vi "File_Update a Path in Keeper.vi"(8 "Error":errorcluster, 9 "File / Directory Name":string, 10 "New Path":path, 11 "INI File Path":path) -> (0 "Error Out":errorcluster)   [LabVIEW 2020]
uses:
  <vilib>/Utility/config.llb/NI_LVConfig.lvlib
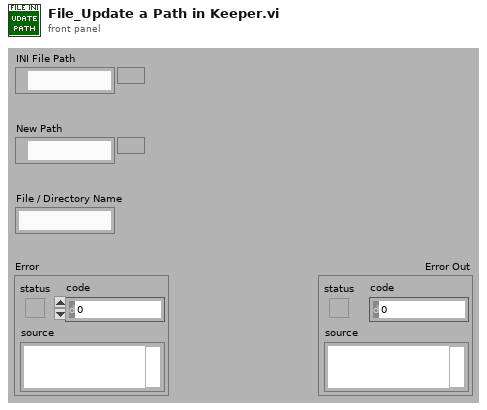
[diagram p1: front panel]
types:
  T1 = typedef "NI_LVConfig.lvlib/Config Data RefNum.ctl" = refnum<k1>
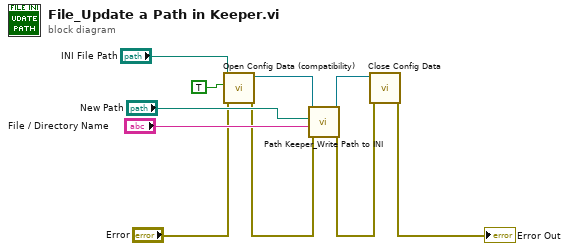
[diagram p0: block diagram]
diagram:
  n1 = call <vilib>:"Open Config Data (compatibility).vi"("error in (no error)"="Error", "create file if necessary (T)"=TRUE ("create file if necessary? (T)"), "configuration file path"="INI File Path") -> ("error out"=w5:errorcluster, "refnum"=w7:T1)  [unwired: 6 in, 1 out]
  n2 = call "Path Keeper_Write Path to INI.vi"("Error In"=w5, "File / Directory Name In"="File / Directory Name", "Path In"="New Path", "Ini Ref In"=w7) -> ("Error Out"=w6:errorcluster, "Ini Ref Out"=w8:T1)  [unwired: 5 in, 1 out]
  n3 = call <vilib>:"Close Config Data.vi"("error in (no error)"=w6, "refnum"=w8) -> ("error out"=→"Error Out":errorcluster)  [unwired: 8 in, 1 out]
